vi "Set Cluster Element by Name.vi"(8 "错误输入":errorcluster, 9 "Element Name(\"\":New Element Data Name)":string, 10 "New Element Value":variant, 11 "Cluster":variant) -> (0 "错误输出":errorcluster, 3 "VCluster out":variant)   [LabVIEW 2012, in "TD Tools.lvlib"]
uses:
  TD Tools.lvlib
panel:
  out "found?":bool
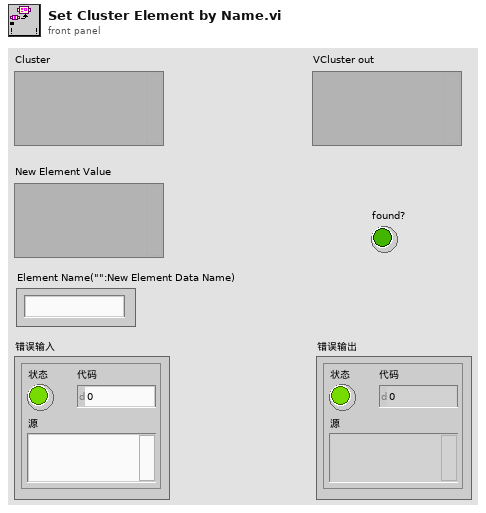
[diagram p1: front panel]
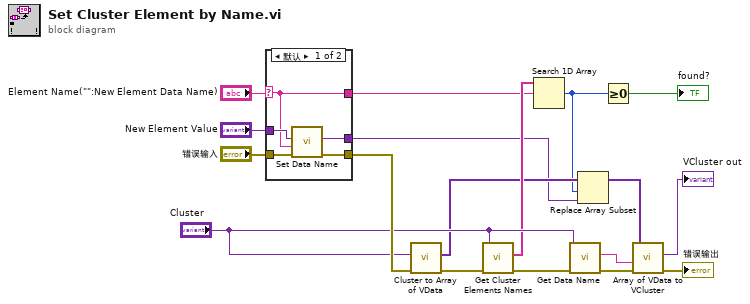
[diagram p0: block diagram]
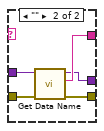
[diagram p2: hidden frame]
diagram:
  n1 = case shown="默认" "Element Name(\"\":New Element Data Name)" {
    selector: "Element Name(\"\":New Element Data Name)" -> [w22 _]
    tunnel: "错误输入" -> [w19 w27]
    tunnel: [w22 w26] -> w10
    tunnel: "New Element Value" -> [w23 w24]
    tunnel: [w21 w24] -> w6
    tunnel: [w20 w25] -> w15
    frame Default {
      n2 = call "Set Data Name.vi"("错误输入"=w19, "Data Name"=w22, "Data"=w23) -> ("错误输出"=w20:errorcluster, "Renamed Data"=w21:variant)  [unwired: 7 in]
    }
    frame "" {
      n3 = call "Get Data Name.vi"("错误输入"=w27, "Data"=w24) -> ("错误输出"=w25:errorcluster, "Data Name"=w26:string)  [unwired: 7 in, 1 out]
    }
  }
  n4 = call "Cluster to Array of VData.vi"("错误输入"=w15, "Cluster"="Cluster") -> ("错误输出"=w14:errorcluster, "Array of VData"=w8:variant[])  [unwired: 8 in]
  n5 = call "Get Cluster Elements Names.vi"("错误输入"=w14, "Cluster"="Cluster") -> ("错误输出"=w13:errorcluster, "Elements Names"=w11:string[])  [unwired: 8 in]
  n6 = Search 1D Array(1D array=w11, element=w10) -> (index of element=w7:i32)  [unwired: 1 in]
  n7 = call "Get Data Name.vi"("错误输入"=w13, "Data"="Cluster") -> ("错误输出"=w1:errorcluster, "Data Name"=w4:string)  [unwired: 7 in, 1 out]
  n8 = Replace Array Subset(array=w8, new element=w6, index=w7) -> (w5:variant[])
  n9 = Greater Or Equal To 0?(x=w7) -> (x >= 0?=→"found?":bool)
  n10 = call "Array of VData to VCluster.vi"("error in (no error)"=w1, "Cluster Name"=w4, "Array"=w5) -> ("error out"=→"错误输出":errorcluster, "VCluster"=→"VCluster out":variant)  [unwired: 7 in]
